vi "MOVING OBJECTS.vi"() -> ()   [LabVIEW 2018]
panel:
  out "String":string
  in  "Numeric":dbl
  in  "Slide":dbl(slide) scale=100.0..-100.0
  in  "Boolean":bool
  in  "stop":bool
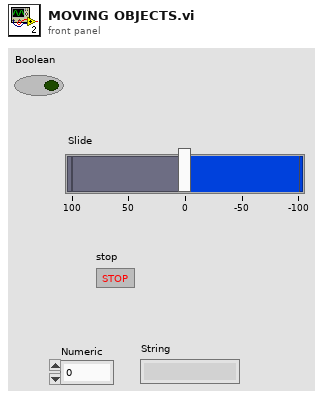
[diagram p1: front panel]
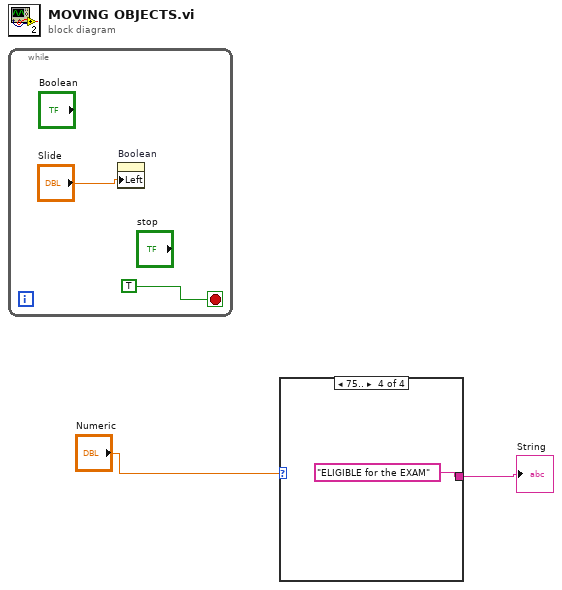
[diagram p0: block diagram]
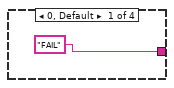
[diagram p2: hidden frame]
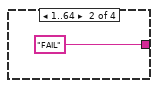
[diagram p3: hidden frame]
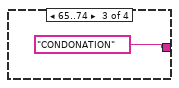
[diagram p4: hidden frame]
diagram:
  n1 = while {
    stop <- TRUE stop-if-true
    n2 = property on="Boolean" class="Bool (strict)"("Left"="Slide") -> ()  [unwired: 2 in, 2 out]
  }
  n3 = case shown="75.." "Numeric" {
    tunnel: ["FAIL" "FAIL" "CONDONATION" "ELIGIBLE for the EXAM"] -> w1
    frame 0, Default {
    }
    frame 1..64 {
    }
    frame 65..74 {
    }
    frame 75.. {
    }
  }
  "String" <- w1
